vi "TSPopup.Demo Registration.vi"(0 "TSPopup in":refnum<class "TSPopup.lvclass">, 1 "Signal Settings ref":refnum<vi>, 3 "error in (no error)":errorcluster) -> (7 "TSPopup out":refnum<class "TSPopup.lvclass">, 10 "error out":errorcluster)   [LabVIEW 2016, in "TSPopup.lvlib" / "TSPopup.lvclass"]
doc: "VI to hold all the different type registrations for this specific demo.\n\nType Sensitive Popup \nCopyright © 2007, J. David Saunders\nAll rights reserved."
uses:
  <userlib>/TSPopup/TSPopup.lvclass
  <userlib>/TSPopup/TSPopup.Popup Call Parameters.ctl
  <userlib>/TSPopup/TSPopup.Data Type.ctl
  <vilib>/Utility/miscctls.llb/LVRowAndColumnTypeDef.ctl
panel:
  in  "Active Cell:Active Cell":T1
  in  "Show Popup (type only)":T2
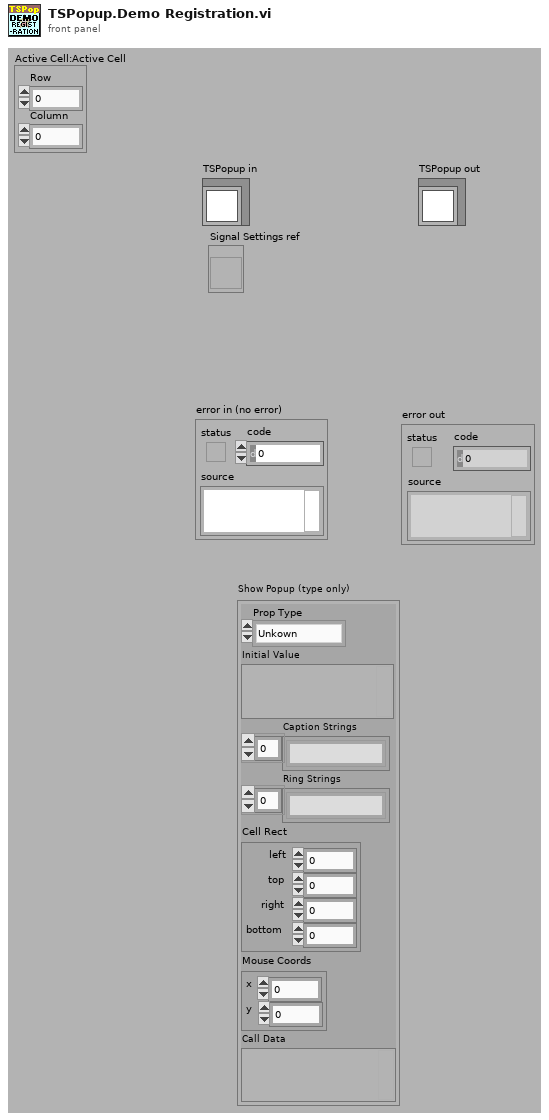
[diagram p1: front panel]
types:
  T1 = typedef "LVRowAndColumnTypeDef.ctl" = cluster{"Row":i32, "Column":i32}
  T2 = typedef "TSPopup.lvlib/TSPopup.lvclass/TSPopup.Popup Call Parameters.ctl" = cluster{"Prop Type":T3, "Initial Value":variant, "Caption Strings":string[], "Ring Strings":string[], "Cell Rect":cluster{"left":i16, "top":i16, "right":i16, "bottom":i16}, "Mouse Coords":cluster{"x":i16, "y":i16}, "Call Data":variant}
  T3 = typedef "TSPopup.lvlib/TSPopup.lvclass/TSPopup.Data Type.ctl" = enum16{"Unkown", "NO POPUP", "String", "Integer", "Float", "Color", "Boolean", "Ring", "Captioned String", "Captioned Integer", "Button Color", "2 Int Cluster", "4 Int Cluster", "check"}
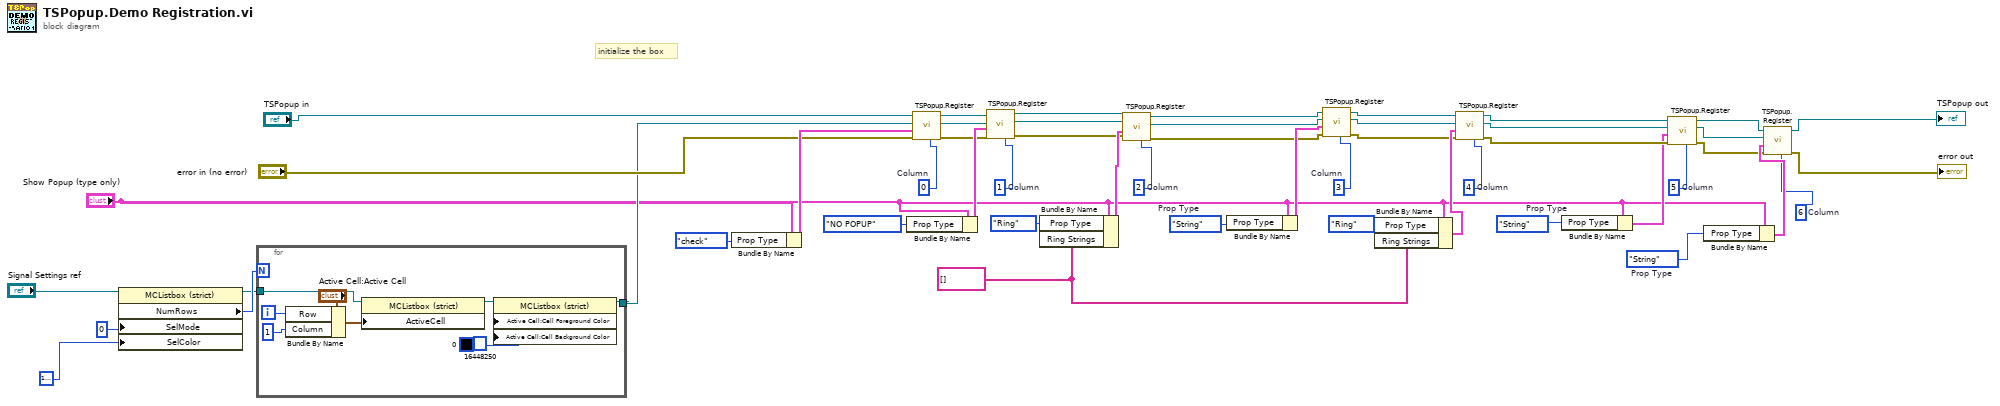
[diagram p0: block diagram]
diagram:
  w1 = 6  # Column
  w7 = TSPopup.Data_Type."String"  # Prop Type
  w12 = string[] [] ("Ring Strings")
  w42 = 0  # Column
  w18 = 5  # Column
  w47 = TSPopup.Data_Type."String"  # Prop Type
  w23 = 4  # Column
  w33 = 2  # Column
  w37 = 1  # Column
  w27 = 3  # Column
  w51 = TSPopup.Data_Type."String"  # Prop Type
  # "initialize the box"
  n1 = property class="MCListbox (strict)"(reference="Signal Settings ref", "SelMode"=u32 0 ("Selection Color"), "SelColor"=u32 16777216) -> (reference out=w15:refnum<vi>, "NumRows"=w16:u32)  [unwired: 1 in, 1 out]
  n2 = for {
    N: w16 -> [_]
    tunnel: w15 -> [w60]
    tunnel: [w58] -> w13
    i -> [w59]
    n3 = Bundle By Name(cluster="Active Cell:Active Cell", "Row"=w59, "Column"=1) -> (w55:T1)
    n4 = property class="MCListbox (strict)"(reference=w60, "ActiveCell"=w55) -> (reference out=w57:refnum<vi>)  [unwired: 1 in, 1 out]
    n5 = property class="MCListbox (strict)"(reference=w57, "Active Cell:Cell Foreground Color"=u32 0, "Active Cell:Cell Background Color"=u32 16448250) -> (reference out=w58:refnum<vi>)  [unwired: 1 in, 1 out]
  }
  n6 = Bundle By Name(cluster="Show Popup (type only)", "Prop Type"=TSPopup.Data_Type."check") -> (w44:T2)
  n7 = Bundle By Name(cluster="Show Popup (type only)", "Prop Type"=TSPopup.Data_Type."NO POPUP") -> (w39:T2)
  n8 = call <userlib>:"TSPopup.Register.vi"("Col (unwired = all columns)"=w42, "error in (no error)"="error in (no error)", "Parameters"=w44, "Ctl Refnum"=w13, "TSPopup in"="TSPopup in") -> ("error out"=w38:errorcluster, "dup ref out"=w40:refnum<vi>, "TSPopup out"=w41:refnum<class "TSPopup.lvclass">)  [unwired: 4 in]
  n9 = call <userlib>:"TSPopup.Register.vi"("Col (unwired = all columns)"=w37, "error in (no error)"=w38, "Parameters"=w39, "Ctl Refnum"=w40, "TSPopup in"=w41) -> ("error out"=w28:errorcluster, "dup ref out"=w35:refnum<vi>, "TSPopup out"=w36:refnum<class "TSPopup.lvclass">)  [unwired: 4 in]
  n10 = Bundle By Name(cluster="Show Popup (type only)", "Prop Type"=TSPopup.Data_Type."Ring", "Ring Strings"=w12) -> (w34:T2)
  n11 = call <userlib>:"TSPopup.Register.vi"("Col (unwired = all columns)"=w33, "error in (no error)"=w28, "Parameters"=w34, "Ctl Refnum"=w35, "TSPopup in"=w36) -> ("error out"=w29:errorcluster, "dup ref out"=w31:refnum<vi>, "TSPopup out"=w32:refnum<class "TSPopup.lvclass">)  [unwired: 4 in]
  n12 = Bundle By Name(cluster="Show Popup (type only)", "Prop Type"=w51) -> (w30:T2)
  n13 = call <userlib>:"TSPopup.Register.vi"("Col (unwired = all columns)"=w27, "error in (no error)"=w29, "Parameters"=w30, "Ctl Refnum"=w31, "TSPopup in"=w32) -> ("error out"=w19:errorcluster, "dup ref out"=w25:refnum<vi>, "TSPopup out"=w26:refnum<class "TSPopup.lvclass">)  [unwired: 4 in]
  n14 = Bundle By Name(cluster="Show Popup (type only)", "Prop Type"=TSPopup.Data_Type."Ring", "Ring Strings"=w12) -> (w24:T2)
  n15 = call <userlib>:"TSPopup.Register.vi"("Col (unwired = all columns)"=w23, "error in (no error)"=w19, "Parameters"=w24, "Ctl Refnum"=w25, "TSPopup in"=w26) -> ("error out"=w20:errorcluster, "dup ref out"=w21:refnum<vi>, "TSPopup out"=w22:refnum<class "TSPopup.lvclass">)  [unwired: 4 in]
  n16 = Bundle By Name(cluster="Show Popup (type only)", "Prop Type"=w47) -> (w17:T2)
  n17 = call <userlib>:"TSPopup.Register.vi"("Col (unwired = all columns)"=w18, "error in (no error)"=w20, "Parameters"=w17, "Ctl Refnum"=w21, "TSPopup in"=w22) -> ("error out"=w5:errorcluster, "dup ref out"=w10:refnum<vi>, "TSPopup out"=w11:refnum<class "TSPopup.lvclass">)  [unwired: 4 in]
  n18 = Bundle By Name(cluster="Show Popup (type only)", "Prop Type"=w7) -> (w6:T2)
  n19 = call <userlib>:"TSPopup.Register.vi"("Col (unwired = all columns)"=w1, "error in (no error)"=w5, "Parameters"=w6, "Ctl Refnum"=w10, "TSPopup in"=w11) -> ("error out"=→"error out":errorcluster, "TSPopup out"=→"TSPopup out":refnum<class "TSPopup.lvclass">)  [unwired: 4 in, 1 out]
